vi "MFCselectionOops.vi"(4 "currentCombo":T3[](array[typedef]), 5 "MFCcapabilities":T3[](array[typedef]), 6 "MdotMin":dbl=nan, 7 "MdotMax":dbl=nan, 9 "Mdot":dbl) -> (0 "OffCentre":dbl, 1 "suggestedCombo":T3[](array[typedef]), 2 "nMFCs":i32)   [LabVIEW 2016]
uses:
  MFCcapability.ctl
  ComboRange.ctl
  MFCselectionData.ctl
  SelectionStages.ctl
panel:
  out "Array":T1[](array[typedef])
  out "Cluster":T2
  out "SuggestedRange":T4
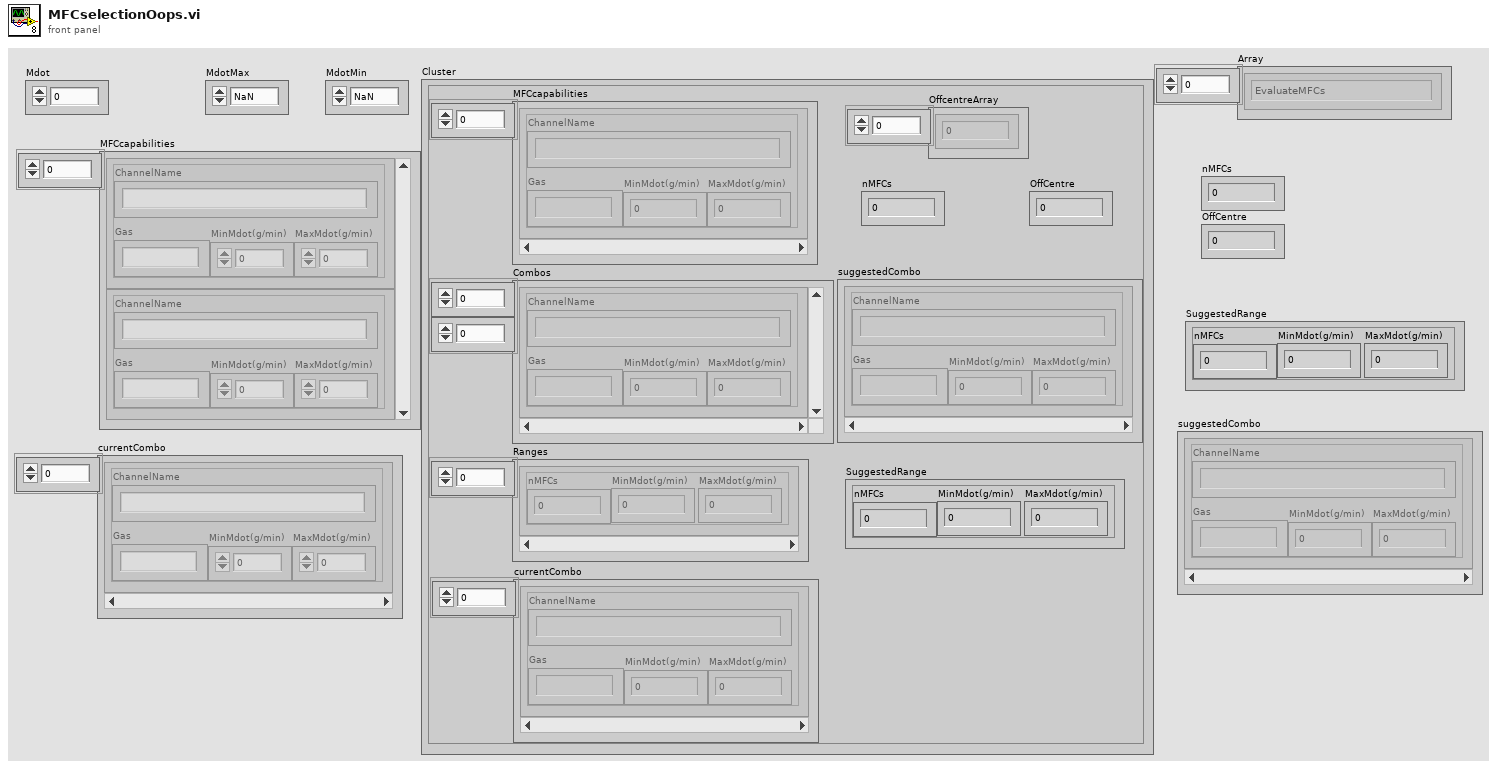
[diagram p1: front panel]
types:
  T1 = typedef "SelectionStages.ctl" = enum16{"EvaluateMFCs", "AccumulateMFCs", "Initialise", "HaveLimits?", "CurrentComboViable?", "CurrentComboRange?", "GetAllCombos", "ExtractViableCombos", "EvaluateViableCombos", "WhatNext?", "ErrorReport", "FinalOutput"}
  T2 = typedef "MFCselectionData.ctl" = cluster{"MFCcapabilities":T3[], "Combos":T3[][], "Ranges":T4[], "OffcentreArray":dbl[], "SuggestedRange":T4, "suggestedCombo":T3[], "OffCentre":dbl, "nMFCs":i32, "currentCombo":T3[]}
  T3 = typedef "MFCcapability.ctl" = cluster{"ChannelName":string, "MinMdot(g/min)":dbl, "MaxMdot(g/min)":dbl, "Gas":string}
  T4 = typedef "ComboRange.ctl" = cluster{"nMFCs":i32, "MinMdot(g/min)":dbl, "MaxMdot(g/min)":dbl}
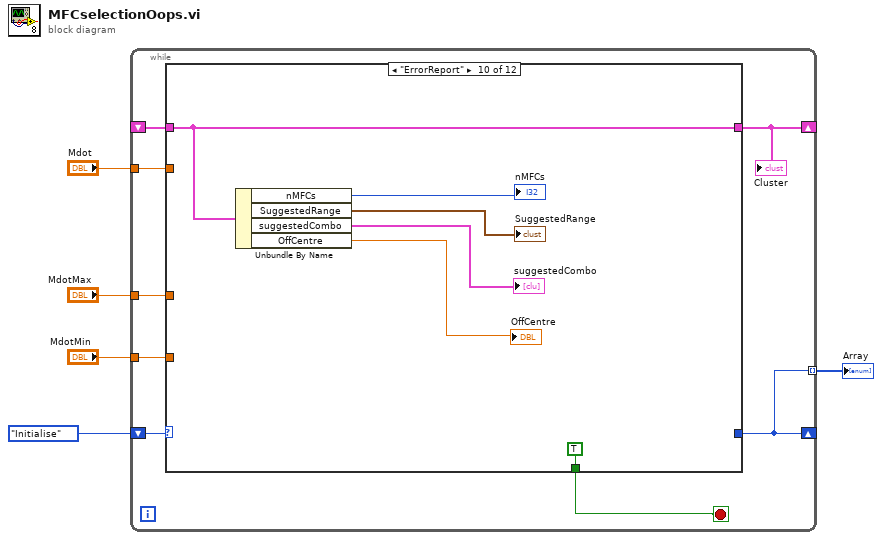
[diagram p0: block diagram]
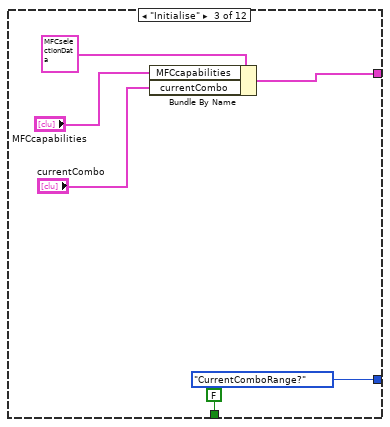
[diagram p4: hidden frame]
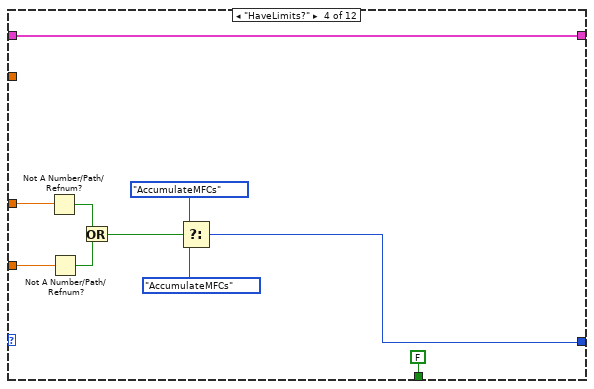
[diagram p5: hidden frame]
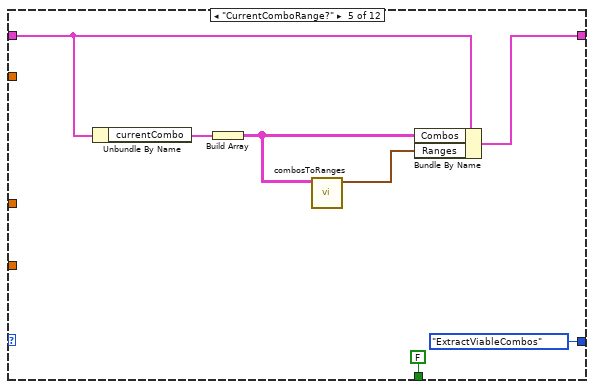
[diagram p6: hidden frame]
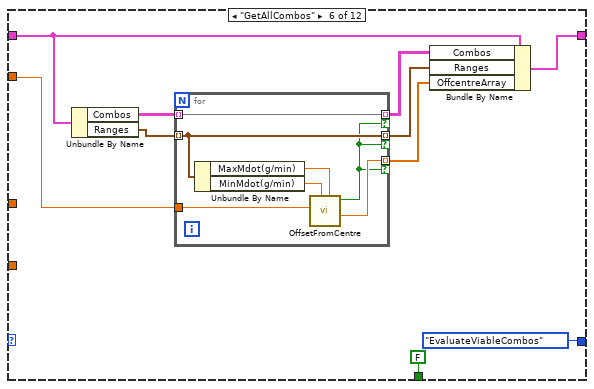
[diagram p7: hidden frame]
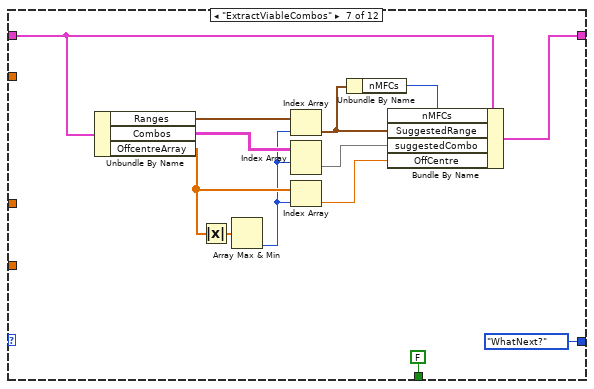
[diagram p8: hidden frame]
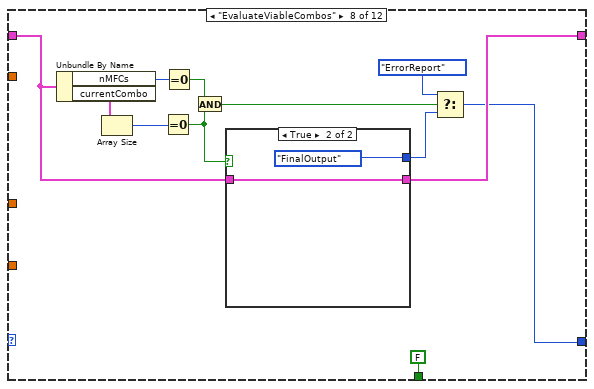
[diagram p9: hidden frame]
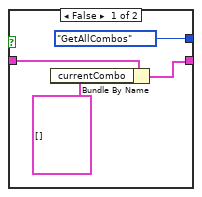
[diagram p10: hidden frame]
diagram:
  n1 = while {
    shift-right: [w6] -> _
    shift-left: SelectionStages."Initialise" -> [w13]
    tunnel: "MdotMax" -> [w12]
    tunnel: "MdotMin" -> [w11]
    tunnel: "Mdot" -> [w10]
    shift-right: [w8] -> _
    shift-left: _ -> [w7]
    tunnel: [w6] -> w1 mode=indexing
    stop <- w9 stop-if-true
    n2 = case shown="\"ErrorReport\"" w13 {
      tunnel: w12 -> [_ _ _ w31 _ _ _ _ _ _ _ _]
      tunnel: w11 -> [_ _ _ w30 _ _ _ _ _ _ _ _]
      tunnel: [_ _ SelectionStages."CurrentComboRange?" w25 SelectionStages."ExtractViableCombos" SelectionStages."EvaluateViableCombos" SelectionStages."WhatNext?" w69 _ _ _ _] -> w6
      tunnel: w10 -> [_ _ _ _ _ w47 _ _ _ _ _ _]
      tunnel: [_ _ FALSE FALSE FALSE FALSE FALSE FALSE _ TRUE _ _] -> w9
      tunnel: [w14 w15 w19 w22 w37 w43 w56 w71 w87 w93 w94 w95] -> w8
      tunnel: w7 -> [w14 w15 _ w22 w33 w44 w57 w72 w87 w93 w94 w95]
      frame "AccumulateMFCs" {
      }
      frame "EvaluateMFCs" {
      }
      frame "Initialise" {
        n3 = Bundle By Name(cluster=T2 {"MFCcapabilities"=[], "Combos"=[], "Ranges"=[], "OffcentreArray"=[], "SuggestedRange"={"nMFCs"=0, "MinMdot(g/min)"=0.0, "MaxMdot(g/min)"=0.0}, "suggestedCombo"=[], "OffCentre"=0.0, "nMFCs"=0, "currentCombo"=[]}, "MFCcapabilities"="MFCcapabilities", "currentCombo"="currentCombo") -> (w19:T2)
      }
      frame "HaveLimits?" {
        n4 = Not A Number/Path/Refnum?(number/path/refnum=w31) -> (NaN/Path/Refnum?=w29:bool)
        n5 = Not A Number/Path/Refnum?(number/path/refnum=w30) -> (NaN/Path/Refnum?=w28:bool)
        n6 = Or(x=w29, y=w28) -> (x .or. y?=w27:bool)
        n7 = Select(t=SelectionStages."AccumulateMFCs", s=w27, f=SelectionStages."AccumulateMFCs") -> (s? t:f=w25:T1)
      }
      frame "CurrentComboRange?" {
        n8 = Unbundle By Name(w33) -> ("currentCombo"=w32:T3[])
        n9 = Build Array(w32) -> (w35:T3[][])
        n10 = call "combosToRanges.vi"("combosIn"=w35) -> ("rangesOut"=w38:T4[])  [unwired: 10 in]
        n11 = Bundle By Name(cluster=w33, "Combos"=w35, "Ranges"=w38) -> (w37:T2)
      }
      frame "GetAllCombos" {
        n12 = Unbundle By Name(w44) -> ("Combos"=w46:T3[][], "Ranges"=w48:T4[])
        n13 = for {
          tunnel: w48 -> [w54] mode=indexing
          tunnel: w47 -> [w51]
          tunnel: [w55] -> w42 mode=indexing if=w49
          tunnel: w46 -> [w55] mode=indexing
          tunnel: [w54] -> w41 mode=indexing if=w49
          tunnel: [w50] -> w40 mode=indexing if=w49
          n14 = Unbundle By Name(w54) -> ("MaxMdot(g/min)"=w52:dbl, "MinMdot(g/min)"=w53:dbl)
          n15 = call "OffsetFromCentre.vi"("RangeMax"=w52, "RangeMin"=w53, "Value"=w51) -> ("OffsetFromCentre"=w50:dbl, "In Range?"=w49:bool)  [unwired: 6 in, 1 out]
        }
        n16 = Bundle By Name(cluster=w44, "Combos"=w42, "Ranges"=w41, "OffcentreArray"=w40) -> (w43:T2)
      }
      frame "ExtractViableCombos" {
        n17 = Unbundle By Name(w57) -> ("Ranges"=w67:T4[], "Combos"=w68:T3[][], "OffcentreArray"=w64:dbl[])
        n18 = Absolute Value(x=w64) -> (abs(x)=w65:dbl[])
        n19 = Array Max & Min(array=w65) -> (min index (indices)=w63:i32)  [unwired: 3 out]
        n20 = Index Array(array=w67, index=w63) -> (element=w60:T4)
        n21 = Index Array(array=w68, index (row)=w63) -> (element=w59:T3[])  [unwired: 1 in]
        n22 = Index Array(array=w64, index=w63) -> (element=w58:dbl)
        n23 = Unbundle By Name(w60) -> ("nMFCs"=w61:i32)
        n24 = Bundle By Name(cluster=w57, "nMFCs"=w61, "SuggestedRange"=w60, "suggestedCombo"=w59, "OffCentre"=w58) -> (w56:T2)
      }
      frame "EvaluateViableCombos" {
        n25 = Unbundle By Name(w72) -> ("nMFCs"=w79:i32, "currentCombo"=w74:T3[])
        n26 = Array Size(array=w74) -> (size(s)=w78:i32)
        n27 = Equal To 0?(x=w78) -> (x = 0?=w73:bool)
        n28 = Equal To 0?(x=w79) -> (x = 0?=w76:bool)
        n29 = And(x=w76, y=w73) -> (x .and. y?=w75:bool)
        n30 = case shown="True" w73 {
          tunnel: [w83 w86] -> w71
          tunnel: w72 -> [w84 w86]
          tunnel: [SelectionStages."GetAllCombos" SelectionStages."FinalOutput"] -> w70
          frame False {
            n31 = Bundle By Name(cluster=w84, "currentCombo"=T3[] []) -> (w83:T2)
          }
          frame True {
          }
        }
        n32 = Select(t=SelectionStages."ErrorReport", s=w75, f=w70) -> (s? t:f=w69:T1)
      }
      frame "WhatNext?" {
      }
      frame "ErrorReport" {
        n33 = Unbundle By Name(w93) -> ("nMFCs"=→"nMFCs":i32, "SuggestedRange"=→"SuggestedRange":T4, "suggestedCombo"=→"suggestedCombo":T3[], "OffCentre"=→"OffCentre":dbl)
      }
      frame "FinalOutput" {
      }
      frame "CurrentComboViable?" {
      }
    }
    "Cluster" <- w8
  }
  "Array" <- w1
